vi "move.vi"(6 "delay before read (ms)":u32=50, 8 "error in (no error)":errorcluster, 9 "Grating, gr/mm":u16(ring)=2 items=["2400", "1800", "1200", "600", "300", "150"], 11 "Wavelength, nm":dbl=10.0 format="%.3f") -> (0 "error out":errorcluster)   [LabVIEW 2017]
doc: "The Advanced Serial Read and Write example performs a Serial Port Read, a Serial Port Write, or a combination of these actions while setting some advanced serial features like buffer size, termination characters, and XON/XOFF flow control. The user selects the actions (read or write) on the front panel. If both are selected, the VI will write the data first, read the data and then close the VISA session that is opened to the port. \n\nThe parameters set for the serial port must match the parameters of the connected instrument or device. In this example, the bytes to read parameter specifies the number of bytes that the serial port reads. If there were more bytes at the port than the number specified in bytes to read, those bytes would not be read. Also, if you specify to read more bytes than the number of bytes actually read, you might receive a timeout error message.\n\nINSTRUCTIONS:\n1) Select the serial resource and configuration parameters (baud rate, data bits, parity, stop bits, flow control).\n2) Termination character can be enabled and set. Also, set the required input buffer size prior to running the example.\n3) Select the operations to be performed. \n4) Connect the serial port to your device. If no device is available, perform a loopback test by doing one of the following. Short pins 2 and 3 on a RS-232 cable or short pin 4 to pin 8 and pin 5 to pin 9 on a RS-485/422 cable. \n5) Run the VI to see the data read. (The \"read string\" will match the \"string to write\" if a loopback test was performed.)\n\nThis example exposes several advanced features that you may need for your application. Not all applications need all the features shown in this example. The input buffer size is likely an important setting that you want to control in your application. This example expands upon the flow control option for XON and XOFF, allowing the user to choose those control characters. The timeout parameter has been brought to the front panel so a user can specify the time period the VISA Read will wait for the number of bytes to read before timing out. Also, the user has several controls for the termination character, which is discussed later.\n\nNote that you can press the write and read buttons and change the bytes to read parameters on the fly, while the example is running. However, you must stop the example to change the other configuration parameters after the example has started running, and then run again.\n\nSet the I/O buffer size slightly higher the amount of data you expect to receive. This is very important for applications that don't use flow control, as you may lose characters if the receive buffer overflows.\n\nSetting the timeout period ensures that the operation returns with a timeout error if the operation cannot be performed in the specified time period. \n\nSome devices require a termination character in order to identify the end of command strings. Some devices send a termination character to signify the end of data to be read. \n\nThis example shows how you can end the Read operation once a termination character is detected in the buffer and/or append a termination character at the end of the Write data. To enable the Read to end on a termination character, use the VISA Configure Serial Port or use the VISA Properties Serial End Mode for Reads, Termination Character Enable, and Termination Character. To end the Write with a termination character, use the VISA Properties Serial End Mode for Writes, the Send End Enable, and Termination Character. In this example, the same termination character is used for both the Read and the Write. You can specify two different characters for your application, if desired.\n\nYour application may require specific characters for the XON/XOFF Flow Control. You can specify these characters with the VISA Properties Flow Control XOFF Character and Flow Control XON Character. Note that if the standard XON and XOFF characters are used, then decimal 17 and 19 are unavailable for data values. Remember that using flow control and setting an adequate buffer size allow you to prevent buffer overflows."
uses:
  Serial comms/Serial comms.lvlib
  Monochromator.lvlib
  <vilib>/Utility/error.llb/DialogType.ctl
panel:
  in  "VISA resource name":refnum<visa-resource-name>="COM1"
  in  "baud rate":u32=9600
  out "move":bool
  out "delay":bool
  out "move done":bool
  out "bytes to read":u32
  out "string 2":string="\n"
  out "Loop":i32
  in  "stop":bool
  # "Move Wavelength"
  # "nm"
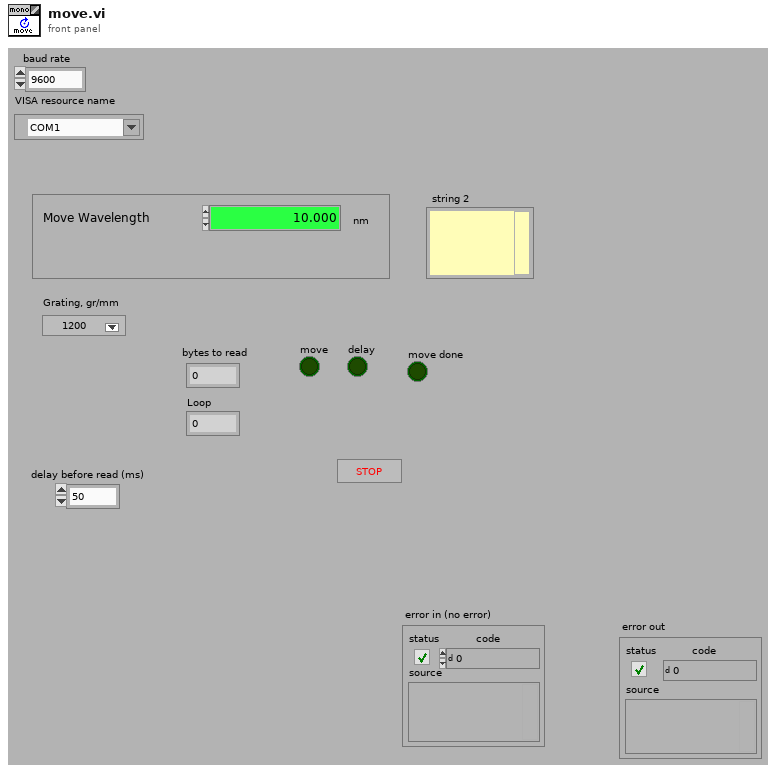
[diagram p1: front panel]
types:
  T1 = typedef "DialogType.ctl" = u16
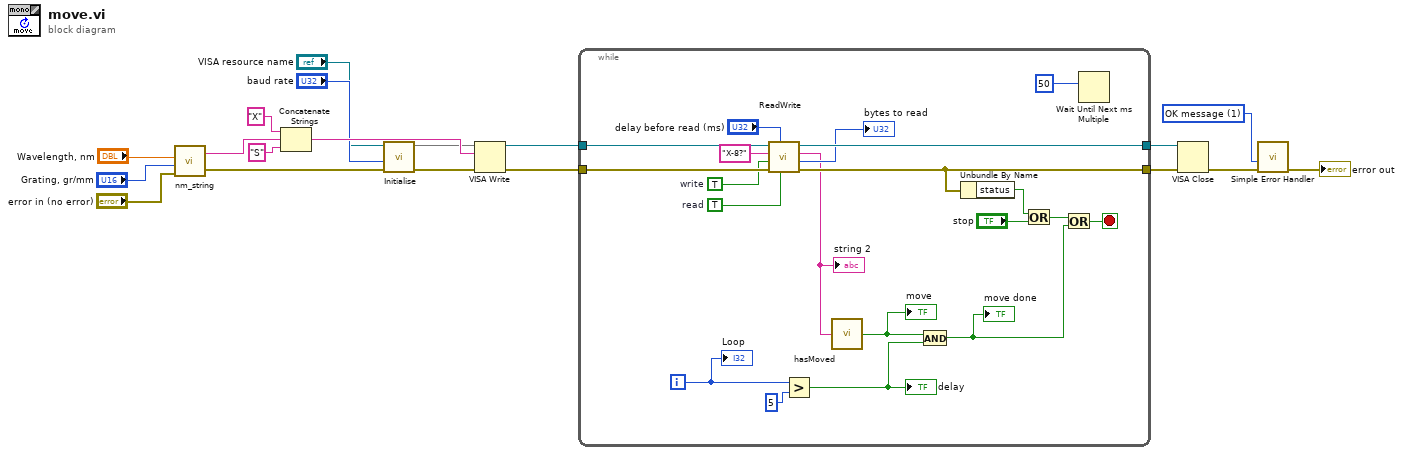
[diagram p0: block diagram]
diagram:
  w13 = T1 1 items=["no dialog", "OK message", "continue or stop message", "OK message + warnings", "continue/stop + warnings"] ("type of dialog (OK msg:1)")
  n1 = call "nm_string.vi"("error in (no error)"="error in (no error)", "Grating, gr/mm"="Grating, gr/mm", "Wavelength, nm"="Wavelength, nm") -> ("error out"=w4:errorcluster, "nm_String"=w10:string)  [unwired: 1 in]
  n2 = Concatenate Strings("X" ("string"), w10, "S" ("string")) -> (w14:string)
  n3 = call "Initialise.vi"("error in"=w4, 9:"baud rate", 11:"VISA resource name") -> ("error out"=w6:errorcluster, 3:w7)  [unwired: 6 in, 1 out]
  n4 = VISA Write(VISA resource name=w7, write buffer=w14, error in (no error)=w6) -> (VISA resource name out=w16:refnum<visa-resource-name>, error out=w15:errorcluster)  [unwired: 1 out]
  n5 = while {
    tunnel: [w39] -> w18
    tunnel: [w38] -> w17
    tunnel: w16 -> [w34]
    tunnel: w15 -> [w33]
    i -> [w25]
    stop <- w31 stop-if-true
    w27 = TRUE  # read
    w29 = TRUE  # write
    n6 = call "ReadWrite.vi"("read"=w27, "delay before read (ms)"="delay before read (ms)", "error in"=w33, "write"=w29, "string to write"="X-8?", "VISA  name in"=w34) -> ("error out"=w38:errorcluster, "bytes to read"=→"bytes to read":u32, "read string"=w23:string, "VISA out"=w39:refnum<visa-resource-name>)
    "string 2" <- w23
    n7 = Greater?(x=w25, y=5 ("x")) -> (0:w20:bool)
    "delay" <- w20
    n8 = call "hasMoved.vi"("read string 2"=w23) -> ("move"=w21:bool)
    "move" <- w21
    n9 = And(x=w21, y=w20) -> (x .and. y?=w22:bool)
    "move done" <- w22
    n10 = Unbundle By Name(w38) -> ("status"=w37:bool)
    n11 = Or(x=w37, y="stop") -> (x .or. y?=w32:bool)
    n12 = Or(x=w32, y=w22) -> (x .or. y?=w31:bool)
    n13 = Wait Until Next ms Multiple(millisecond multiple=u32 50) -> ()  [unwired: 1 out]
    "Loop" <- w25
  }
  n14 = VISA Close(VISA resource name=w18, error in (no error)=w17) -> (error out=w19:errorcluster)
  n15 = call <vilib>:"Simple Error Handler.vi"("type of dialog (OK msg:1)"=w13, "error in (no error)"=w19) -> ("error out"=→"error out":errorcluster)  [unwired: 3 in, 4 out]
